vi "Asylum_EnsureIgorStringFormat.vi"(8 "error in (no error)":errorcluster, 11 "Value":string) -> (0 "error out":errorcluster, 3 "Value":string)   [LabVIEW 2016]
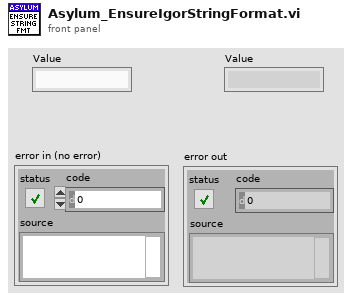
[diagram p1: front panel]
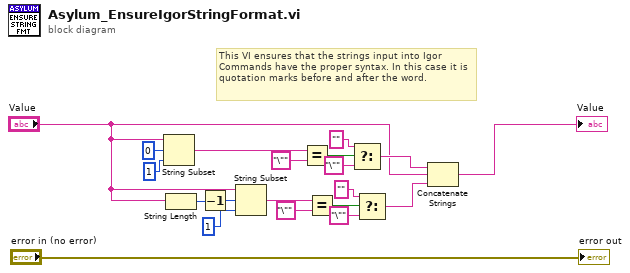
[diagram p0: block diagram]
diagram:
  # "This VI ensures that the strings input into Igor Commands have the proper syntax. In this case it is quotation marks before and after the word."
  n1 = String Subset(string="Value", offset (0)=0, length (rest)=1 ("length (rest)")) -> (substring=w13:string)
  n2 = String Length(string="Value") -> (length=w19:i32)
  n3 = Decrement(x=w19) -> (x-1=w18:i32)
  n4 = String Subset(string="Value", offset (0)=w18, length (rest)=1 ("length (rest)")) -> (substring=w5:string)
  n5 = Equal?(x=w13, y="\"") -> (x = y?=w14:bool)
  n6 = Equal?(x=w5, y="\"") -> (x = y?=w6:bool)
  n7 = Select(t="", s=w14, f="\"") -> (s? t:f=w4:string)
  n8 = Select(t="", s=w6, f="\"") -> (s? t:f=w3:string)
  n9 = Concatenate Strings(w4, "Value", w3) -> (→"Value":string)
  "error out" <- "error in (no error)"
